vi "1_Build_Data_SubVI.vi"(9 "Phase Data":dbl min=0.0 max=360.0 step=1.0, 10 "Frequency Data":dbl min=0.0 max=37500000.0 step=1.0 format="%#_10g", 11 "Waveform Type":T1(ring)) -> (3 "Message":string)   [LabVIEW 2024]
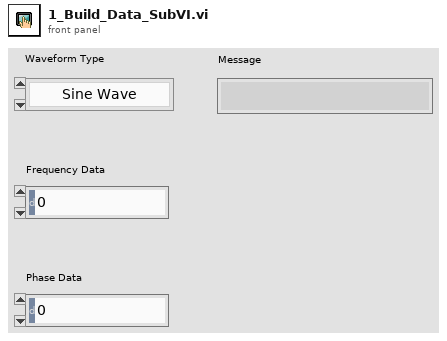
[diagram p1: front panel]
types:
  T1 = enum16{"Sine Wave", "Triangular Wave", "Square Wave"}
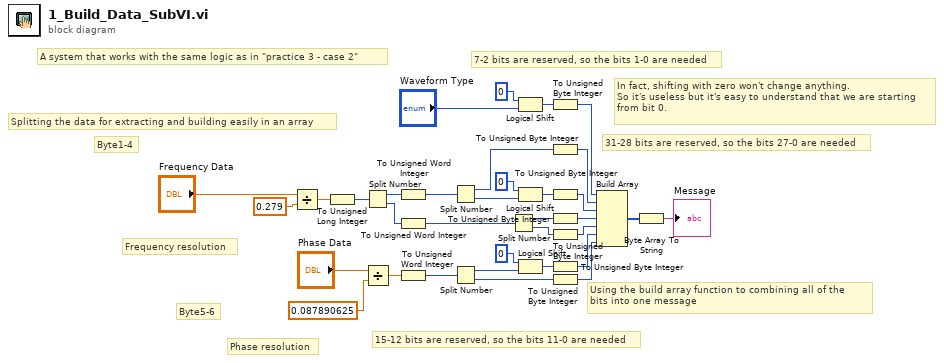
[diagram p0: block diagram]
diagram:
  # "In fact, shifting with zero won't change anything.\nSo it's useless but it's easy to understand that we are starting\nfrom bit 0."
  # "7-2 bits are reserved, so the bits 1-0 are needed"
  # "31-28 bits are reserved, so the bits 27-0 are needed"
  # "Using the build array function to combining all of the\nbits into one message"
  # "15-12 bits are reserved, so the bits 11-0 are needed"
  # "Splitting the data for extracting and building easily in an array"
  # "A system that works with the same logic as in \"practice 3 - case 2\""
  # "Byte5-6"
  # "Byte1-4"
  # "Phase resolution"
  # "Frequency resolution"
  n1 = Divide(x="Frequency Data", y=0.279) -> (x/y=w4:dbl)
  n2 = To Unsigned Long Integer(number=w4) -> (unsigned 32bit integer=w5:u32)
  n3 = Split Number(x=w5) -> (hi(x)=w6:u16, lo(x)=w7:u16)
  n4 = Divide(x="Phase Data", y=0.087890625) -> (x/y=w14:dbl)
  n5 = To Unsigned Word Integer(number=w6) -> (unsigned 16bit integer=w8:u16)
  n6 = To Unsigned Word Integer(number=w7) -> (unsigned 16bit integer=w9:u16)
  n7 = To Unsigned Word Integer(number=w14) -> (unsigned 16bit integer=w15:u16)
  n8 = Split Number(x=w8) -> (hi(x)=w1:u8, lo(x)=w17:u8)
  n9 = Split Number(x=w15) -> (hi(x)=w19:u8, lo(x)=w25:u8)
  n10 = Split Number(x=w9) -> (hi(x)=w22:u8, lo(x)=w23:u8)
  n11 = Logical Shift(y=i16 0, x="Waveform Type") -> (x << y=w20:u32)
  n12 = Logical Shift(y=i16 0, x=w17) -> (x << y=w21:u8)
  n13 = Logical Shift(y=i16 0, x=w19) -> (x << y=w24:u8)
  n14 = To Unsigned Byte Integer(number=w20) -> (unsigned 8bit integer=w26:u8)
  n15 = To Unsigned Byte Integer(number=w1) -> (unsigned 8bit integer=w27:u8)
  n16 = To Unsigned Byte Integer(number=w21) -> (unsigned 8bit integer=w28:u8)
  n17 = To Unsigned Byte Integer(number=w22) -> (unsigned 8bit integer=w29:u8)
  n18 = To Unsigned Byte Integer(number=w23) -> (unsigned 8bit integer=w30:u8)
  n19 = To Unsigned Byte Integer(number=w24) -> (unsigned 8bit integer=w31:u8)
  n20 = To Unsigned Byte Integer(number=w25) -> (unsigned 8bit integer=w32:u8)
  n21 = Build Array "Build Array"(w26, w27, w28, w29, w30, w31, w32) -> (w33:u8[])
  n22 = Byte Array To String(unsigned byte array=w33) -> (string=→"Message":string)
